vi "Parameter.vi"(8 "error in (no error)":errorcluster caption="entrée d'erreur (pas d'erreur)", 10 "Parameter":T1, 11 "Actor_EventStart en entrée":refnum<class "Actor_EventStart.lvclass">) -> (0 "error out":errorcluster caption="sortie d'erreur", 3 "Actor_EventStart en sortie":refnum<class "Actor_EventStart.lvclass">)   [LabVIEW 2020, in "Library Core.lvlib" / "Actor_EventStart.lvlib" / "Actor_EventStart.lvclass"]
uses:
  Actor_EventStart.lvclass
  Instrument/Instrument (Default)/Class Instrument (Default).lvclass
  Classe Event (Default)/Class Event (Default).lvclass
  Commun VI/TypeDef/Variable Printable.ctl
  Actor_EventStart.lvclass/Actor_EventStart.ctl
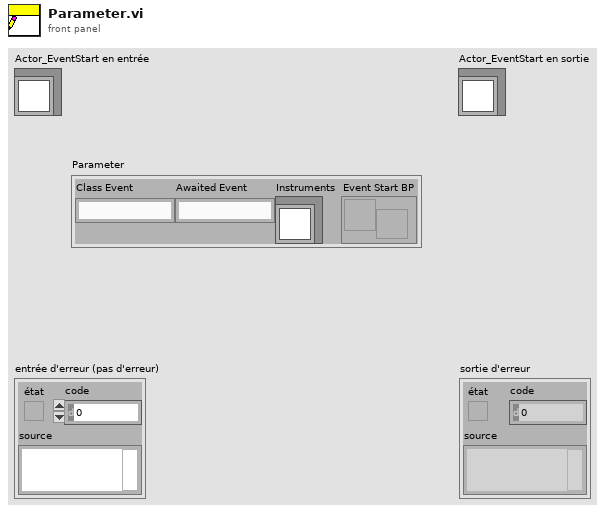
[diagram p1: front panel]
types:
  T1 = cluster{"Class Event":string, "Awaited Event":string, "Instruments":refnum<class "Class Instrument (Default).lvclass">, "Event Start BP":refnum<user-event>}
  T2 = enum16{"Get Variable", "Get All Variables", "Set Variable", "Delete Variable", "Delete All Variable"}
  T3 = typedef "Variable Printable.ctl" = string
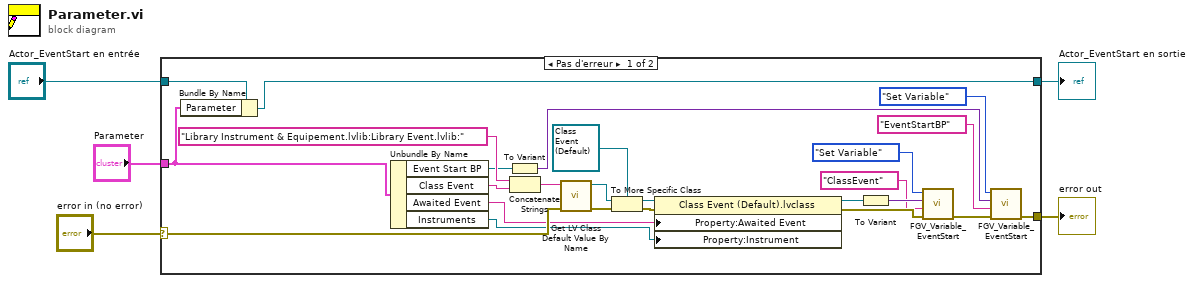
[diagram p0: block diagram]
diagram:
  n1 = case shown="Pas d'erreur" "error in (no error)" {
    selector: "error in (no error)" -> [w25 w31]
    tunnel: [w8 w31] -> w4
    tunnel: [w29 w32] -> w2
    tunnel: "Actor_EventStart en entrée" -> [w30 w32]
    tunnel: "Parameter" -> [w28 _]
    frame No Error {
      n2 = Bundle By Name(cluster=w30, "Parameter"=w28) -> (w29:refnum<class "Actor_EventStart.lvclass">)
      n3 = Unbundle By Name(w28) -> ("Event Start BP"=w7:refnum<user-event>, "Class Event"=w18:string, "Awaited Event"=w22:string, "Instruments"=w21:refnum<class "Class Instrument (Default).lvclass">)
      n4 = To Variant(anything=w7) -> (Variant=w6:variant)
      n5 = Concatenate Strings("Library Instrument & Equipement.lvlib:Library Event.lvlib:", w18) -> (w17:string)
      n6 = call <vilib>:"Get LV Class Default Value By Name.vi"("error in (no error)"=w25, "class name"=w17) -> ("error out"=w27:errorcluster, "object"=w26:refnum<class>)  [unwired: 8 in]
      n7 = To More Specific Class(target class=refnum<class "Class Event (Default).lvclass"> refnum ("Library Sequencer.lvlib:Actor_EventStart.lvlib:Class Event (Default).lvclass"), reference=w26, error in=w27) -> (specific class reference=w23:refnum<class "Class Event (Default).lvclass">, error out=w20:errorcluster)
      n8 = property class="Class Event (Default).lvclass"(reference=w23, error in=w20, "Property:Awaited Event"=w22, "Property:Instrument"=w21) -> (reference out=w14:refnum<class "Class Event (Default).lvclass">, error out=w16:errorcluster)
      n9 = To Variant(anything=w14) -> (Variant=w15:variant)
      n10 = call "FGV_Variable_EventStart.vi"("error in (no error)"=w16, "Variable"=T3 "ClassEvent", "Data In"=w15, "Function"=T2."Set Variable") -> ("error out"=w9:errorcluster)  [unwired: 5 in, 2 out]
      n11 = call "FGV_Variable_EventStart.vi"("error in (no error)"=w9, "Variable"=T3 "EventStartBP", "Data In"=w6, "Function"=T2."Set Variable") -> ("error out"=w8:errorcluster)  [unwired: 5 in, 2 out]
    }
    frame Error {
    }
  }
  "error out" <- w4
  "Actor_EventStart en sortie" <- w2
